vi "BracePLUS_Serial_Logger.vi"(10 "Serial Settings":T1={"baud rate"=115200, "data bits"=8, "parity"=enum."None", "stop bits"=10, "flow control"=0} {"flow control" items=["None"=0, "XON/XOFF"=1, "RTS/CTS"=2, "DTR/DSR"=4]; "stop bits" items=["1.0"=10, "1.5"=15, "2.0"=20]; "data bits" min=5 max=8 step=1; "baud rate" items=["75"=75, "110"=110, "134"=134, "150"=150, "300"=300, "600"=600, "1200"=1200, "1800"=1800, "2400"=2400, "4800"=4800, "7200"=7200, "9600"=9600, "14400"=14400, "19200"=19200, "28800"=28800, "38400"=38400, "56000"=56000, "57600"=57600, "115200"=115200, "128000"=128000, "230400"=230400]}, 11 "VISA resource name":refnum<visa-resource-name>="COM16") -> (0 "error out":errorcluster, 3 "Filename":string)   [LabVIEW 2018]
panel:
  in  "Tab Control":enum32{"Display", "Configuration"}(tab)
  out "Elapsed Time (ms)":i16(slide) scale=0.0..110.0
  out "Connected":bool
  out "Initialised":bool
  out "Recording":bool
  out "Init string":string
  # "ESCAPES:Logger"
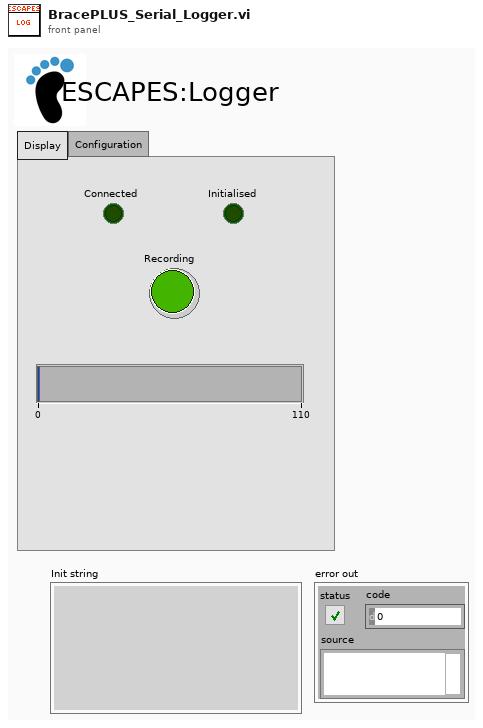
[diagram p1: front panel]
types:
  T1 = cluster{"baud rate":u32, "data bits":u16, "parity":enum16{"None", "Odd", "Even", "Mark", "Space"}, "stop bits":u16, "flow control":u16}
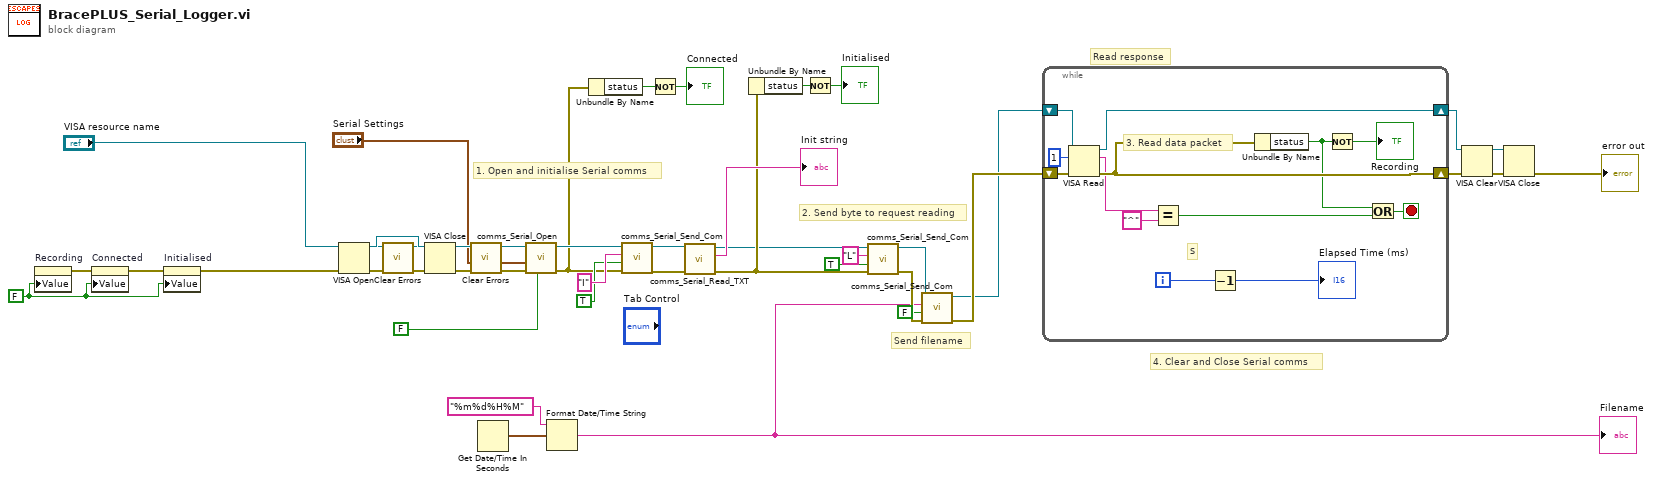
[diagram p0: block diagram]
diagram:
  w21 = FALSE ("Send Init Comm?")
  # "Send filename"
  # "2. Send byte to request reading"
  # "Read response"
  # "4. Clear and Close Serial comms"
  # "1. Open and initialise Serial comms"
  n1 = property on="Recording" class="Bool (strict)"("Value"=w21) -> (error out=w22:errorcluster)  [unwired: 2 in, 1 out]
  n2 = property on="Connected" class="Bool (strict)"(error in=w22, "Value"=w21) -> (error out=w23:errorcluster)  [unwired: 1 in, 1 out]
  n3 = property on="Initialised" class="Bool (strict)"(error in=w23, "Value"=w21) -> (error out=w10:errorcluster)  [unwired: 1 in, 1 out]
  n4 = VISA Open(error in (no error)=w10, VISA resource name="VISA resource name") -> (VISA resource name=w20:refnum<visa-resource-name>, error out=w19:errorcluster)  [unwired: 3 in]
  n5 = call <vilib>:"Clear Errors.vi"("error in (no error)"=w19) -> ("error out"=w18:errorcluster)  [unwired: 5 in, 1 out]
  n6 = VISA Close(VISA resource name=w20, error in (no error)=w18) -> (error out=w17:errorcluster)
  n7 = call <vilib>:"Clear Errors.vi"("error in (no error)"=w17) -> ("error out"=w16:errorcluster)  [unwired: 5 in, 1 out]
  n8 = Get Date/Time In Seconds() -> (seconds since 1Jan1904=w4:timestamp)
  n9 = call "comms_Serial_Open.vi"("Send Init Comm?"=FALSE, "error in (no error)"=w16, "Serial Settings in"="Serial Settings", "VISA Refnum in"="VISA resource name") -> ("error out"=w29:errorcluster, "VISA Refnum out"=w33:refnum<visa-resource-name>)  [unwired: 5 in, 1 out]
  n10 = Format Date/Time String(time format string (%c)="%m%d%H%M", seconds (now)=w4) -> (date/time string=w3:string)  [unwired: 1 in]
  "Filename" <- w3
  n11 = Unbundle By Name(w29) -> ("status"=w28:bool)
  n12 = call "comms_Serial_Send_Com.vi"("Buffer Clear?"=TRUE, "Command"="I", "VISA resource in"=w33) -> ("VISA resource Out"=w31:refnum<visa-resource-name>)  [unwired: 6 in, 2 out]
  n13 = Not(x=w28) -> (.not. x?=→"Connected":bool)
  n14 = call "comms_Serial_Read_TXT.vi"("error in"=w29, "VISA resource in"=w31) -> ("error out"=w26:errorcluster, "Data Out"=→"Init string":string, "VISA resource Out"=w15:refnum<visa-resource-name>)  [unwired: 6 in, 1 out]
  n15 = Unbundle By Name(w26) -> ("status"=w27:bool)
  n16 = Not(x=w27) -> (.not. x?=→"Initialised":bool)
  n17 = call "comms_Serial_Send_Com.vi"("error in"=w26, "Buffer Clear?"=TRUE, "Command"="L", "VISA resource in"=w15) -> ("error out"=w9:errorcluster, "VISA resource Out"=w6:refnum<visa-resource-name>)  [unwired: 5 in, 1 out]
  n18 = call "comms_Serial_Send_Com.vi"("error in"=w9, "Buffer Clear?"=FALSE, "Command"=w3, "VISA resource in"=w6) -> ("error out"=w8:errorcluster, "VISA resource Out"=w5:refnum<visa-resource-name>)  [unwired: 5 in, 1 out]
  n19 = while {
    shift-right: [w50] -> w36
    shift-left: w5 -> [w41]
    shift-right: [w48] -> w35
    shift-left: w8 -> [w51]
    i -> [w47]
    stop <- w43 stop-if-true
    # "3. Read data packet"
    # "S"
    n20 = VISA Read(VISA resource name=w41, byte count=u32 1, error in (no error)=w51) -> (VISA resource name out=w50:refnum<visa-resource-name>, read buffer=w46:string, error out=w48:errorcluster)  [unwired: 1 out]
    n21 = Equal?(x=w46, y="^") -> (x = y?=w44:bool)
    n22 = Decrement(x=w47) -> (x-1=→"Elapsed Time (ms)":i32)
    n23 = Unbundle By Name(w48) -> ("status"=w42:bool)
    n24 = Not(x=w42) -> (.not. x?=→"Recording":bool)
    n25 = Or(x=w42, y=w44) -> (x .or. y?=w43:bool)
  }
  n26 = VISA Clear(VISA resource name=w36, error in (no error)=w35) -> (VISA resource name out=w38:refnum<visa-resource-name>, error out=w37:errorcluster)
  n27 = VISA Close(VISA resource name=w38, error in (no error)=w37) -> (error out=→"error out":errorcluster)
